vi "Read From XML File(string).vi"(8 "error in (no error)":errorcluster, 11 "XML File Path":path) -> (0 "error out":errorcluster, 2 "XML Elements":string, 3 "XML File Path(duplicate)":path)   [LabVIEW 2020]
doc: "Reads and parses tags from a LabVIEW XML file. When you place this VI on the block diagram, the polymorphic VI selector is visible. Use this selector to choose which polymorphic instance to use. All XML data must follow the standard LabVIEW XML schema."
panel:
  in  "Prompt":string="Select Path to XML File"
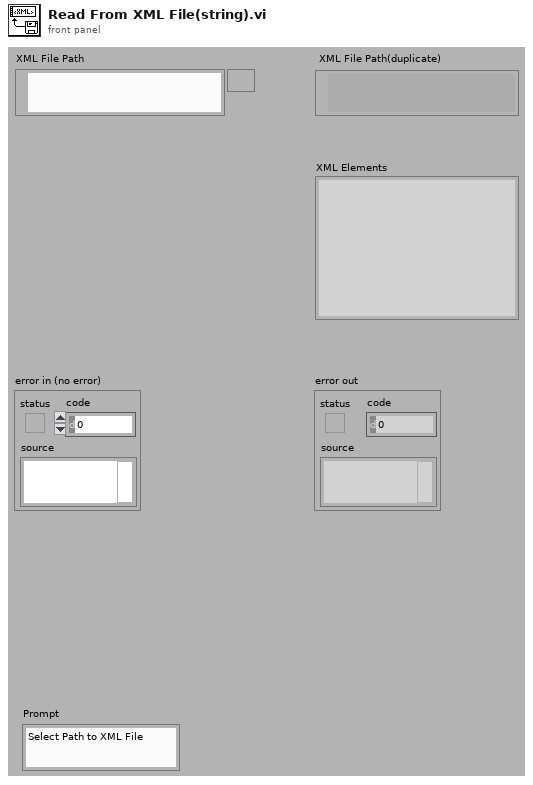
[diagram p1: front panel]
types:
  T1 = enum16{"open", "open or create", "create or replace", "create", "open (read only)"}
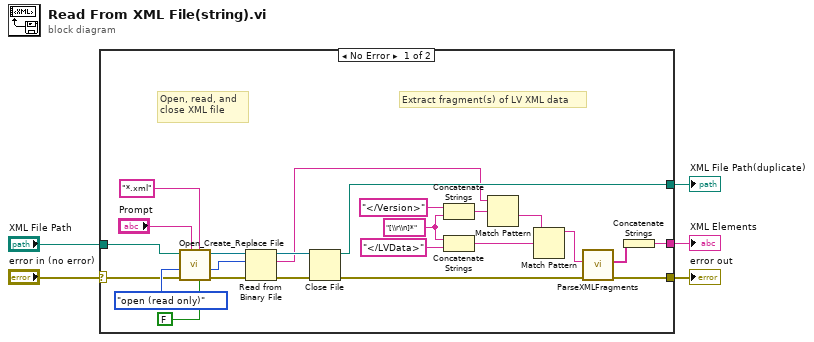
[diagram p0: block diagram]
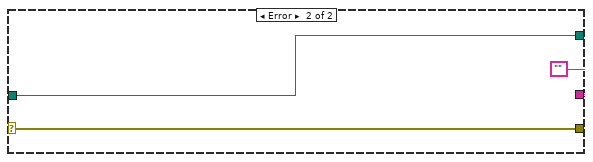
[diagram p2: hidden frame]
diagram:
  n1 = case shown="No Error" "error in (no error)" {
    selector: "error in (no error)" -> [w25 w32]
    tunnel: [w18 w32] -> w4
    tunnel: [w16 w31] -> w3
    tunnel: "XML File Path" -> [w27 w31]
    tunnel: [w14 ""] -> w1
    frame No Error {
      w8 = "[\\r\\n]*"
      # "Extract fragment(s) of LV XML data"
      # "Open, read, and \nclose XML file"
      n2 = call "Open_Create_Replace File.vi"("advisory dialog? (display:T)"=FALSE, "pattern"="*.xml", "prompt"="Prompt", "error in (no error)"=w25, "function (open:0)"=T1."open (read only)", "file path"=w27) -> ("error out"=w11:errorcluster, "file size (bytes)"=w12:i32, "refnum"=w13:refnum<file>)  [unwired: 2 in, 1 out]
      n3 = Read from Binary File(8:w11, 10:w12, 11:w13) -> (0:w9:errorcluster, 2:w7:string, 3:w10:refnum<file>)  [unwired: 3 in, 1 out]
      n4 = Close File(refnum=w10, error in=w9) -> (path=w16:path, error out=w17:errorcluster)
      n5 = Concatenate Strings("</Version>", w8) -> (w20:string)
      n6 = Concatenate Strings(w8, "</LVData>" ("Substring")) -> (w21:string)
      n7 = Match Pattern(string=w7, regular expression=w20) -> (after substring=w22:string)  [unwired: 1 in, 3 out]
      n8 = Match Pattern(string=w22, regular expression=w21) -> (before substring=w19:string)  [unwired: 1 in, 3 out]
      n9 = call "ParseXMLFragments.vi"("error in (no error)"=w17, "XML in"=w19) -> ("error out"=w18:errorcluster, "XML Elements"=w15:string[])  [unwired: 8 in]
      n10 = Concatenate Strings(w15) -> (w14:string)
    }
    frame Error {
    }
  }
  "error out" <- w4
  "XML File Path(duplicate)" <- w3
  "XML Elements" <- w1
